vi "Get num array.vi"(11 "number String":string) -> (3 "number Array":i64[](array[numeric]))   [LabVIEW 2023]
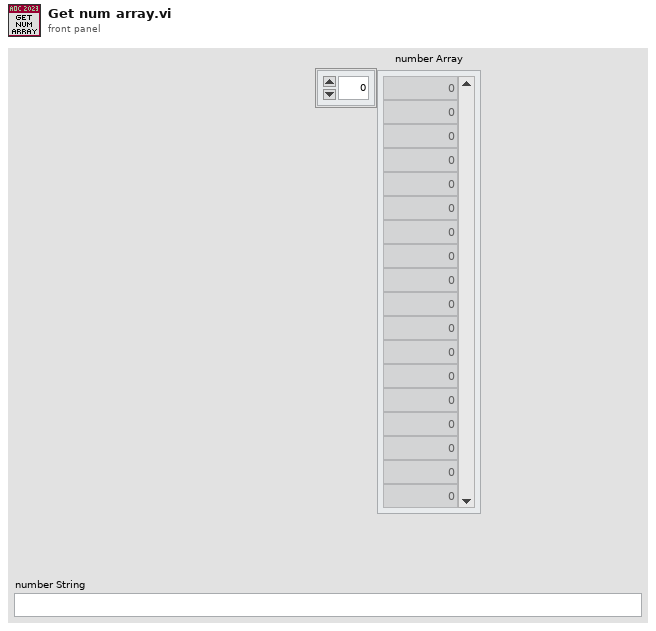
[diagram p1: front panel]
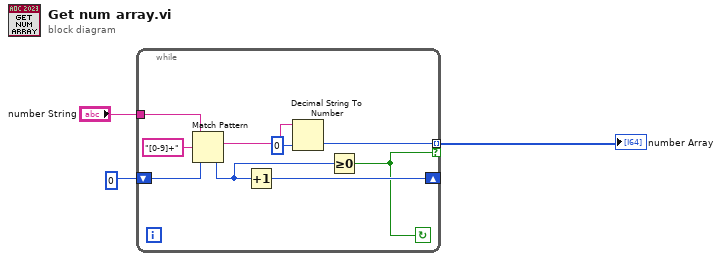
[diagram p0: block diagram]
diagram:
  n1 = while {
    tunnel: "number String" -> [w12]
    shift-right: [w9] -> _
    shift-left: 0 -> [w10]
    tunnel: [w5] -> w1 mode=indexing if=w7
    stop <- w7 continue-if-true
    n2 = Match Pattern(string=w12, regular expression="[0-9]+", offset (0)=w10) -> (match substring=w6:string, offset past match=w8:i32)  [unwired: 2 out]
    n3 = Increment(x=w8) -> (x+1=w9:i32)
    n4 = Decimal String To Number(string=w6, default (0L)=i64 0 ("default (0 I32)")) -> (number=w5:i64)  [unwired: 1 in, 1 out]
    n5 = Greater Or Equal To 0?(x=w8) -> (x >= 0?=w7:bool)
  }
  "number Array" <- w1
